vi "Get Header String.vi"(8 "error in (no error)":errorcluster, 11 "Cookie in":refnum<class "Cookie.lvclass">) -> (0 "error out":errorcluster, 2 "Header String":string, 3 "Cookie out":refnum<class "Cookie.lvclass">)   [LabVIEW 2020, in "HTTP Utils.lvlib" / "Cookie.lvclass"]
uses:
  Cookie.lvclass
  Cookie.lvclass/Cookie.ctl
  HTTP Utils.lvlib
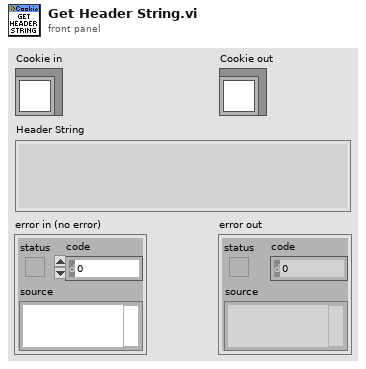
[diagram p1: front panel]
types:
  T1 = typedef "HTTP Utils.lvlib/Cookie Prefix.ctl" = enum16{"None", "Host", "Secure"}
  T2 = typedef "HTTP Utils.lvlib/Cookie SameSite.ctl" = enum16{"Unset (Lax)", "Lax", "Strict", "None"}
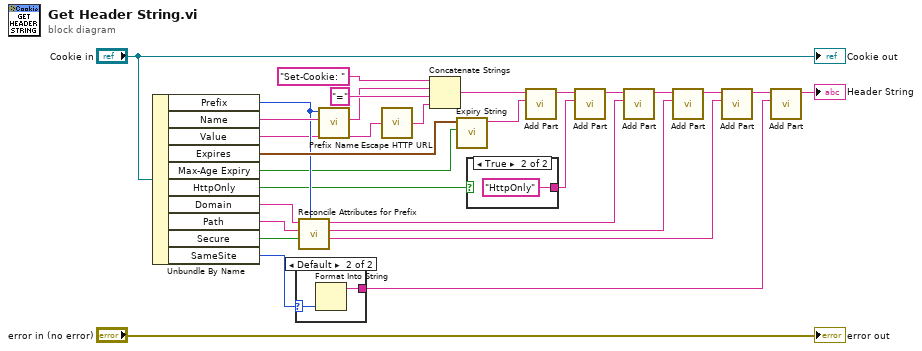
[diagram p0: block diagram]
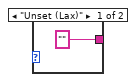
[diagram p2: hidden frame]
diagram:
  n1 = Unbundle By Name("Cookie in") -> ("Prefix"=w16:T1, "Name"=w24:string, "Value"=w3:string, "Expires"=w27:timestamp, "Max-Age Expiry"=w1:bool, "HttpOnly"=w9:bool, "Domain"=w18:string, "Path"=w19:string, "Secure"=w17:bool, "SameSite"=w7:T2)
  n2 = case shown="Default" w7 {
    selector: w7 -> [_ w32]
    tunnel: ["" w31] -> w5
    frame "Unset (Lax)" {
    }
    frame Default {
      n3 = Format Into String(w32) -> (resulting string=w31:string)  [unwired: 3 in, 1 out]
    }
  }
  n4 = call "Reconcile Attributes for Prefix.vi"("Prefix"=w16, "Secure In"=w17, "Path In"=w19, "Domain In"=w18) -> ("Secure"=w10:string, "Path"=w11:string, "Domain"=w12:string)  [unwired: 5 in]
  n5 = call "Prefix Name.vi"("Name"=w24, "Prefix"=w16) -> ("Prefixed Name"=w23:string)  [unwired: 9 in]
  n6 = call "Escape HTTP URL.vi"("unescaped string in"=w3) -> ("escaped string out"=w2:string)
  n7 = Concatenate Strings("Set-Cookie: " ("string"), w23, "=" ("string"), w2) -> (w22:string)
  n8 = call "Expiry String.vi"("As Max-Age? (T)"=w1, "Time Stamp"=w27) -> ("String"=w21:string)  [unwired: 8 in, 1 out]
  n9 = case shown="True" w9 {
    tunnel: [_ "HttpOnly" ("string")] -> w8
    frame False {
    }
    frame True {
    }
  }
  n10 = call "Add Part.vi"("New Portion"=w21, "String In"=w22) -> ("String"=w20:string)  [unwired: 9 in]
  n11 = call "Add Part.vi"("New Portion"=w8, "String In"=w20) -> ("String"=w15:string)  [unwired: 9 in]
  n12 = call "Add Part.vi"("New Portion"=w12, "String In"=w15) -> ("String"=w14:string)  [unwired: 9 in]
  n13 = call "Add Part.vi"("New Portion"=w11, "String In"=w14) -> ("String"=w13:string)  [unwired: 9 in]
  n14 = call "Add Part.vi"("New Portion"=w10, "String In"=w13) -> ("String"=w6:string)  [unwired: 9 in]
  n15 = call "Add Part.vi"("New Portion"=w5, "String In"=w6) -> ("String"=→"Header String":string)  [unwired: 9 in]
  "error out" <- "error in (no error)"
  "Cookie out" <- "Cookie in"
